vi "Memory.Pointer.Swap.Unsafe.vi"(8 "error in (no error)":errorcluster, 10 "pointer b":refnum<class "Memory.Pointer.lvclass">, 11 "pointer a":refnum<class "Memory.Pointer.lvclass">) -> (0 "error out":errorcluster, 2 "pointer b":refnum<class "Memory.Pointer.lvclass">, 3 "pointer a":refnum<class "Memory.Pointer.lvclass">)   [LabVIEW 2016, in "Memory Manager.lvlib" / "Memory.Pointer.lvclass"]
doc: "Swaps the address of the two provided <b>pointers</b>.\n\n<b>Note:</b> This VI is <b>unsafe</b>.\n\nUnsafe means that this function does not evaluate the size parameter of <b>pointer a</b> and <b>pointer b</b> before peforming a memory read/write. Reading/writing more data to a pointer than it has allocated can corrupt or crash LabVIEW."
uses:
  Memory.Pointer.lvclass
  Memory.Pointer.lvclass/Memory.Pointer.ctl
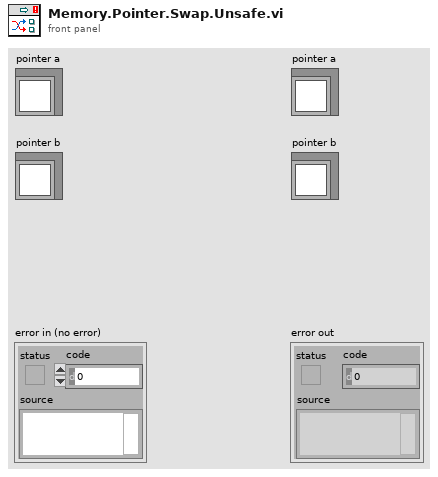
[diagram p1: front panel]
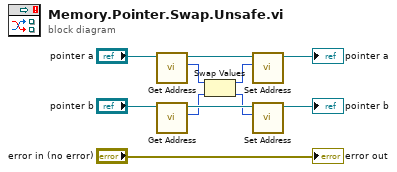
[diagram p0: block diagram]
diagram:
  n1 = call "Get Address.vi"("Pointer in"="pointer a") -> ("address"=w9:u64, "Pointer out"=w7:refnum<class "Memory.Pointer.lvclass">)  [unwired: 8 in, 1 out]
  n2 = call "Get Address.vi"("Pointer in"="pointer b") -> ("address"=w6:u64, "Pointer out"=w8:refnum<class "Memory.Pointer.lvclass">)  [unwired: 8 in, 1 out]
  n3 = Swap Values(12:w9, 14:w6) -> (1:w4:u64, 3:w5:u64)  [unwired: 1 in]
  n4 = call "Set Address.vi"("address"=w4, "Pointer in"=w7) -> ("Pointer out"=→"pointer a":refnum<class "Memory.Pointer.lvclass">)  [unwired: 8 in, 1 out]
  n5 = call "Set Address.vi"("address"=w5, "Pointer in"=w8) -> ("Pointer out"=→"pointer b":refnum<class "Memory.Pointer.lvclass">)  [unwired: 8 in, 1 out]
  "error out" <- "error in (no error)"
